vi "get path to CoreEngine dll.vi"() -> (6 "path to c_interface_calib_vc100.dll":path, 8 "path to c_interface_vc100.dll":path, 10 "path to imoptif":path, 12 "Release/Debug":string)   [LabVIEW 2020]
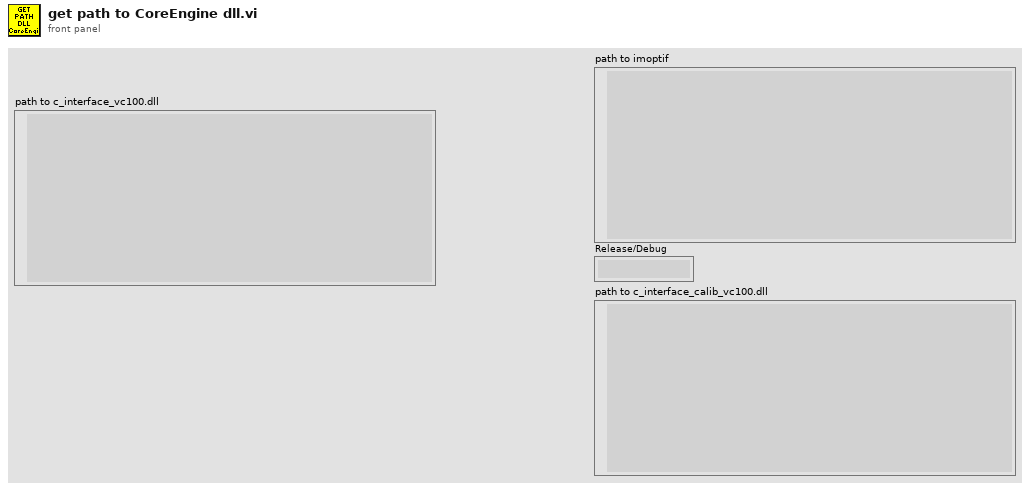
[diagram p1: front panel]
types:
  T1 = enum32{"invalid app kind", "Development System", "Run Time System", "Student Edition", "Embedded LabVIEW", "Evaluation", "Custom"}
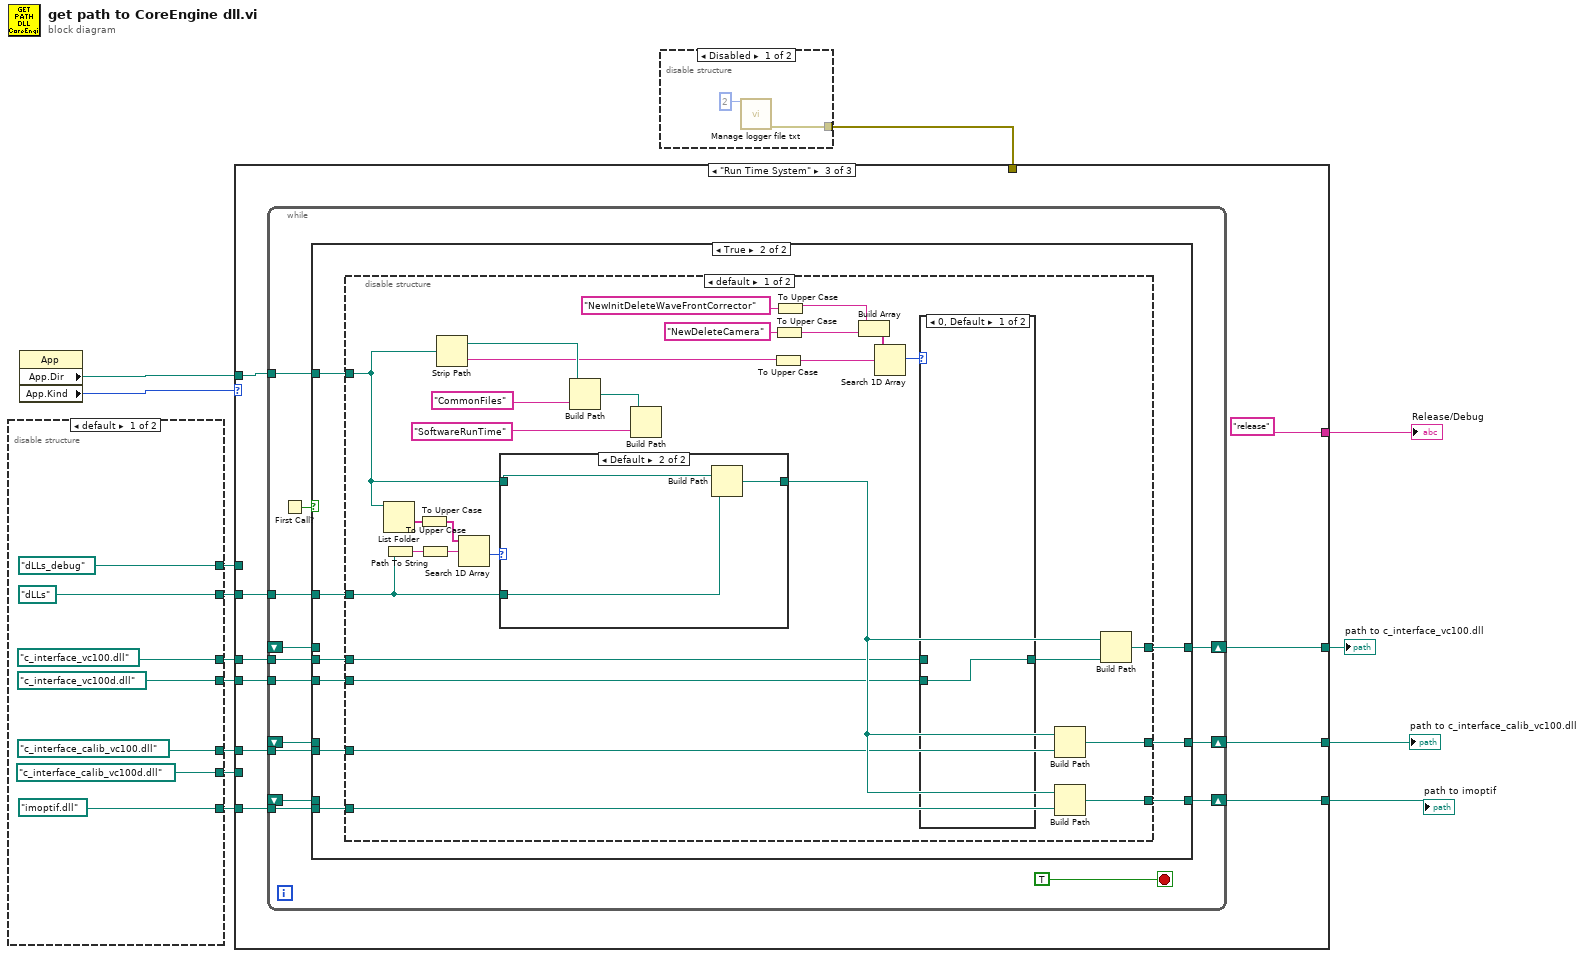
[diagram p0: block diagram]
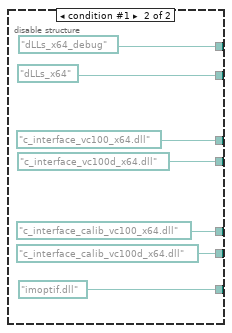
[diagram p3: hidden frame]
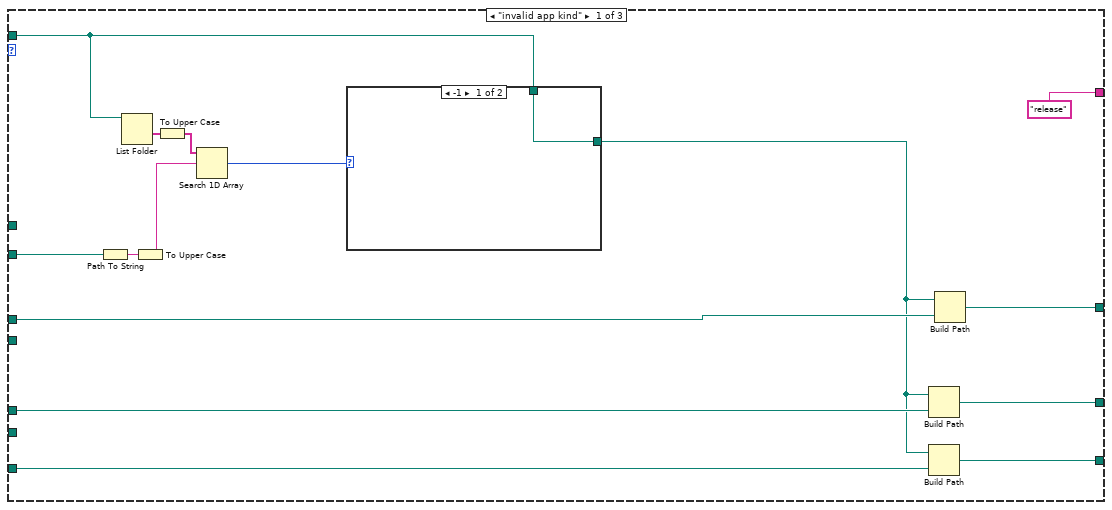
[diagram p4: hidden frame]
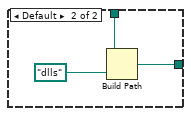
[diagram p5: hidden frame]
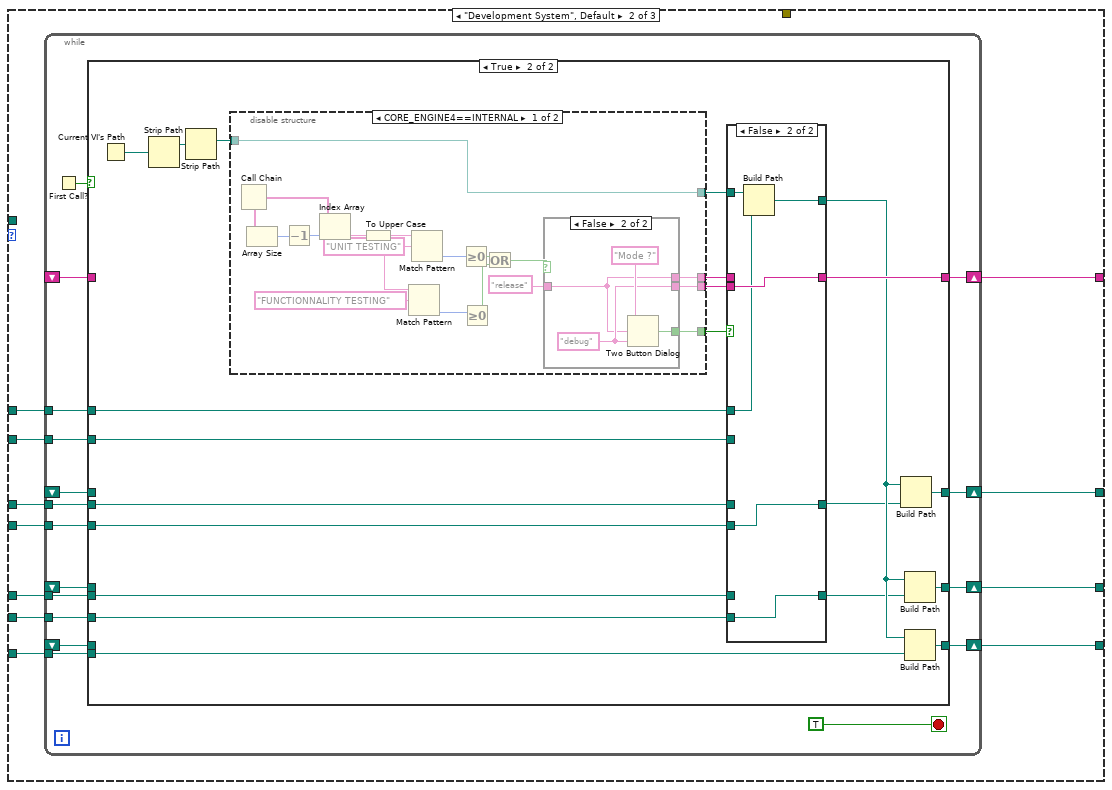
[diagram p6: hidden frame]
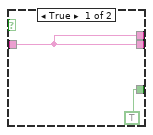
[diagram p8: hidden frame]
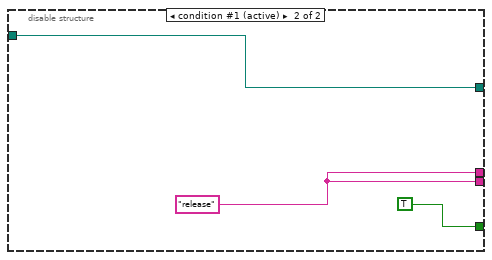
[diagram p9: hidden frame]
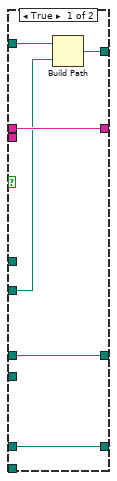
[diagram p10: hidden frame]
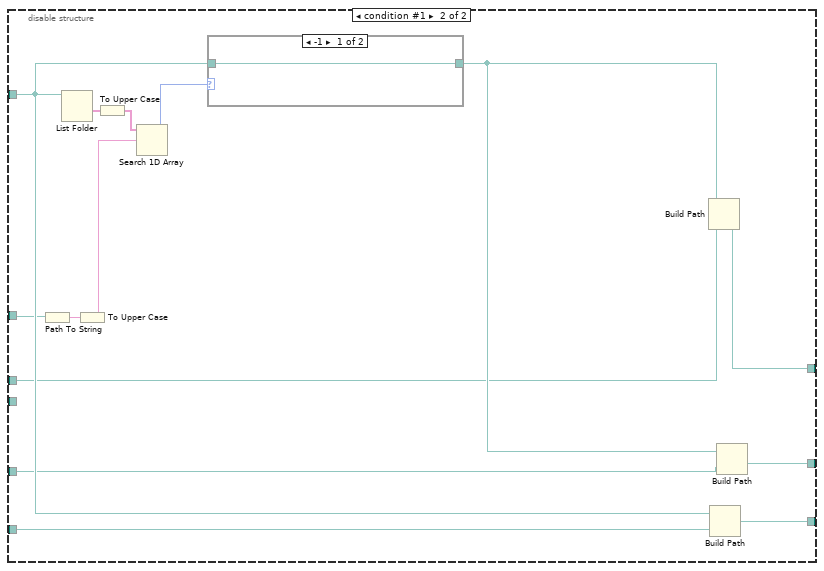
[diagram p14: hidden frame]
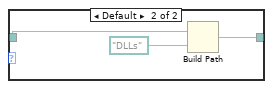
[diagram p15: hidden frame]
diagram:
  n1 = disable-structure shown="default" {
    disable-tunnel: [path "imoptif.dll" ("path in") path "imoptif.dll" ("path in")] -> w13
    disable-tunnel: [path "c_interface_vc100.dll" ("path in") path "c_interface_vc100_x64.dll" ("path in")] -> w8
    disable-tunnel: [path "c_interface_calib_vc100.dll" ("path in") path "c_interface_calib_vc100_x64.dll" ("path in")] -> w7
    disable-tunnel: [path "dLLs" ("path in") path "dLLs_x64" ("path in")] -> w5
    disable-tunnel: [path "dLLs_debug" ("path in") path "dLLs_x64_debug" ("path in")] -> w4
    disable-tunnel: [path "c_interface_vc100d.dll" ("path in") path "c_interface_vc100d_x64.dll" ("path in")] -> w3
    disable-tunnel: [path "c_interface_calib_vc100d.dll" ("path in") path "c_interface_calib_vc100d_x64.dll" ("path in")] -> w2
    frame condition #0 (active) {
    }
    frame condition #1 {
    }
  }
  n2 = property class="App"() -> ("App.Dir"=w10:path, "App.Kind"=w14:T1)  [unwired: 2 in, 2 out]
  n3 = disable-structure shown="Disabled" {
    disable-tunnel: [w29 _] -> w1
    frame Disabled {
      n4 = call "Manage logger file txt.vi"("length"=2) -> ("error out"=w29:errorcluster)  [unwired: 14 in]
    }
    frame Enabled {
    }
  }
  n5 = case shown="\"Run Time System\"" w14 {
    tunnel: [w45 w59 w150] -> w9
    tunnel: w10 -> [w41 _ w147]
    tunnel: w13 -> [w44 w58 w149]
    tunnel: [w43 w57 w148] -> w12
    tunnel: ["release" ("T button name (\"OK\")") w60 "release" ("T button name (\"OK\")")] -> w11
    tunnel: w8 -> [w37 w56 w144]
    tunnel: w7 -> [w36 w55 w143]
    tunnel: [w34 w54 w145] -> w6
    tunnel: w5 -> [w31 w53 w142]
    tunnel: w4 -> [_ w52 _]
    tunnel: w3 -> [_ w51 w141]
    tunnel: w2 -> [_ w50 _]
    tunnel: w1 -> [_ _ _]
    frame "invalid app kind" {
      n6 = Path To String(path=w31) -> (string=w33:string)
      n7 = List Folder(path=w41) -> (folder names=w40:string[])  [unwired: 3 in, 3 out]
      n8 = To Upper Case(1:w33) -> (0:w32:string)
      n9 = To Upper Case(1:w40) -> (0:w38:string[])
      n10 = Search 1D Array(1D array=w38, element=w32) -> (index of element=w39:i32)  [unwired: 1 in]
      n11 = case shown="-1" w39 {
        tunnel: [w46 w48] -> w35
        tunnel: w41 -> [w46 w47]
        frame -1 {
        }
        frame Default {
          n12 = Build Path(base path=w47, name or relative path=path "dlls" ("path in")) -> (appended path=w48:path)
        }
      }
      n13 = Build Path(base path=w35, name or relative path=w36) -> (appended path=w34:path)
      n14 = Build Path(base path=w35, name or relative path=w44) -> (appended path=w43:path)
      n15 = Build Path(base path=w35, name or relative path=w37) -> (appended path=w45:path)
    }
    frame "Development System", Default {
      n16 = while {
        shift-right: [w76] -> w59
        shift-left: _ -> [w75]
        shift-right: [w73] -> w60
        shift-left: _ -> [w72]
        shift-right: [w70] -> w57
        shift-left: _ -> [w69]
        tunnel: w58 -> [w71]
        tunnel: w56 -> [w68]
        tunnel: w55 -> [w67]
        shift-right: [w66] -> w54
        shift-left: _ -> [w65]
        tunnel: w53 -> [w64]
        tunnel: w52 -> [w63]
        tunnel: w51 -> [w62]
        tunnel: w50 -> [w61]
        stop <- TRUE stop-if-true
        n17 = First Call?() -> (First Call?: T/F=w77:bool)
        n18 = case shown="True" w77 {
          tunnel: [w81 w98] -> w76
          tunnel: w75 -> [w81 _]
          tunnel: [w80 w100] -> w73
          tunnel: w72 -> [w80 _]
          tunnel: w71 -> [_ w96]
          tunnel: [w79 w97] -> w70
          tunnel: w69 -> [w79 _]
          tunnel: w68 -> [_ w87]
          tunnel: w67 -> [_ w84]
          tunnel: [w78 w93] -> w66
          tunnel: w65 -> [w78 _]
          tunnel: w64 -> [_ w89]
          tunnel: w63 -> [_ w88]
          tunnel: w62 -> [_ w85]
          tunnel: w61 -> [_ w82]
          frame False {
          }
          frame True {
            n19 = Current VI's Path() -> (path=w94:path)
            n20 = Strip Path(path=w94) -> (stripped path=w95:path)  [unwired: 1 out]
            n21 = Strip Path(path=w95) -> (stripped path=w90:path)  [unwired: 1 out]
            n22 = disable-structure shown="CORE_ENGINE4==INTERNAL" {
              disable-tunnel: [w119 TRUE ("T button?")] -> w102
              disable-tunnel: [w118 w127] -> w101
              disable-tunnel: [w117 w127] -> w99
              disable-tunnel: [w103 w126] -> w92
              disable-tunnel: w90 -> [w103 w126]
              frame condition #0 {
                n23 = Call Chain() -> (call chain=w116:string[])
                n24 = Array Size(array=w116) -> (size(s)=w115:i32)
                n25 = Decrement(x=w115) -> (x-1=w114:i32)
                n26 = Index Array(array=w116, index=w114) -> (element=w113:string)
                n27 = To Upper Case(1:w113) -> (0:w110:string)
                n28 = Match Pattern(string=w110, regular expression="FUNCTIONNALITY TESTING") -> (offset past match=w107:i32)  [unwired: 1 in, 3 out]
                n29 = Match Pattern(string=w110, regular expression="UNIT TESTING") -> (offset past match=w108:i32)  [unwired: 1 in, 3 out]
                n30 = Greater Or Equal To 0?(x=w108) -> (x >= 0?=w106:bool)
                n31 = Greater Or Equal To 0?(x=w107) -> (x >= 0?=w105:bool)
                n32 = Or(x=w106, y=w105) -> (x .or. y?=w104:bool)
                n33 = case shown="False" w104 {
                  tunnel: [TRUE ("T button?") w125] -> w119
                  tunnel: [w121 w122] -> w118
                  tunnel: [w121 w123] -> w117
                  tunnel: "release" ("T button name (\"OK\")") -> [w121 w122]
                  frame True {
                  }
                  frame False {
                    w123 = "debug" ("F button name (\"Cancel\")")
                    n34 = Two Button Dialog(message="Mode ?", 1:w123, 2:w122) -> (T button?=w125:bool)
                  }
                }
              }
              frame condition #1 (active) {
                w127 = "release" ("T button name (\"OK\")")
              }
            }
            n35 = case shown="False" w102 {
              tunnel: [w134 w140] -> w100
              tunnel: w101 -> [w134 _]
              tunnel: w99 -> [_ w140]
              tunnel: w92 -> [w133 w139]
              tunnel: [w132 w138] -> w91
              tunnel: w89 -> [w131 _]
              tunnel: w88 -> [_ w137]
              tunnel: w87 -> [w130 _]
              tunnel: [w130 w136] -> w86
              tunnel: w85 -> [_ w136]
              tunnel: w84 -> [w129 _]
              tunnel: [w129 w135] -> w83
              tunnel: w82 -> [_ w135]
              frame True {
                n36 = Build Path(base path=w133, name or relative path=w131) -> (appended path=w132:path)
              }
              frame False {
                n37 = Build Path(base path=w139, name or relative path=w137) -> (appended path=w138:path)
              }
            }
            n38 = Build Path(base path=w91, name or relative path=w86) -> (appended path=w98:path)
            n39 = Build Path(base path=w91, name or relative path=w83) -> (appended path=w93:path)
            n40 = Build Path(base path=w91, name or relative path=w96) -> (appended path=w97:path)
          }
        }
      }
    }
    frame "Run Time System" {
      n41 = while {
        shift-right: [w163] -> w150
        shift-left: _ -> [w162]
        shift-right: [w159] -> w148
        shift-left: _ -> [w158]
        tunnel: w149 -> [w160]
        tunnel: w147 -> [w157]
        shift-right: [w154] -> w145
        shift-left: _ -> [w153]
        tunnel: w144 -> [w156]
        tunnel: w143 -> [w155]
        tunnel: w142 -> [w152]
        tunnel: w141 -> [w151]
        stop <- TRUE stop-if-true
        n42 = First Call?() -> (First Call?: T/F=w164:bool)
        n43 = case shown="True" w164 {
          tunnel: [w167 w176] -> w163
          tunnel: w162 -> [w167 _]
          tunnel: w160 -> [_ w174]
          tunnel: [w166 w173] -> w159
          tunnel: w158 -> [w166 _]
          tunnel: w157 -> [_ w175]
          tunnel: w156 -> [_ w172]
          tunnel: w155 -> [_ w171]
          tunnel: [w165 w170] -> w154
          tunnel: w153 -> [w165 _]
          tunnel: w152 -> [_ w169]
          tunnel: w151 -> [_ w168]
          frame False {
          }
          frame True {
            n44 = disable-structure shown="default" {
              disable-tunnel: [w204 w224] -> w176
              disable-tunnel: w175 -> [w198 w220]
              disable-tunnel: w174 -> [w200 w219]
              disable-tunnel: [w199 w218] -> w173
              disable-tunnel: w172 -> [w177 w214]
              disable-tunnel: w171 -> [w192 w215]
              disable-tunnel: [w191 w217] -> w170
              disable-tunnel: w169 -> [w182 w212]
              disable-tunnel: w168 -> [w179 _]
              frame condition #0 (active) {
                n45 = List Folder(path=w198) -> (folder names=w203:string[])  [unwired: 3 in, 3 out]
                n46 = Path To String(path=w182) -> (string=w181:string)
                n47 = To Upper Case(1:w203) -> (0:w202:string[])
                n48 = To Upper Case(1:w181) -> (0:w180:string)
                n49 = Strip Path(path=w198) -> (stripped path=w197:path, name=w190:string)
                n50 = Search 1D Array(1D array=w202, element=w180) -> (index of element=w201:i32)  [unwired: 1 in]
                n51 = case shown="Default" w201 {
                  tunnel: [w207 w210] -> w193
                  tunnel: w198 -> [w207 w209]
                  tunnel: w182 -> [_ w208]
                  frame -1 {
                  }
                  frame Default {
                    n52 = Build Path(base path=w209, name or relative path=w208) -> (appended path=w210:path)
                  }
                }
                n53 = Build Path(base path=w197, name or relative path="CommonFiles" ("element")) -> (appended path=w195:path)
                n54 = Build Path(base path=w195, name or relative path="SoftwareRunTime" ("element")) -> ()  [unwired: 1 out]
                n55 = To Upper Case(1:w190) -> (0:w184:string)
                n56 = To Upper Case(1:"NewDeleteCamera" ("element")) -> (0:w186:string)
                n57 = To Upper Case(1:"NewInitDeleteWaveFrontCorrector" ("element")) -> (0:w187:string)
                n58 = Build Array(w187, w186) -> (w185:string[])
                n59 = Search 1D Array(1D array=w185, element=w184) -> (index of element=w183:i32)  [unwired: 1 in]
                n60 = case shown="0, Default" w183 {
                  tunnel: [w205 w206] -> w178
                  tunnel: w179 -> [w205 _]
                  tunnel: w177 -> [_ w206]
                  frame 0, Default {
                  }
                  frame -1 {
                  }
                }
                n61 = Build Path(base path=w193, name or relative path=w192) -> (appended path=w191:path)
                n62 = Build Path(base path=w193, name or relative path=w200) -> (appended path=w199:path)
                n63 = Build Path(base path=w193, name or relative path=w178) -> (appended path=w204:path)
              }
              frame condition #1 {
                n64 = Path To String(path=w212) -> (string=w213:string)
                n65 = List Folder(path=w220) -> (folder names=w223:string[])  [unwired: 3 in, 3 out]
                n66 = To Upper Case(1:w213) -> (0:w211:string)
                n67 = To Upper Case(1:w223) -> (0:w222:string[])
                n68 = Search 1D Array(1D array=w222, element=w211) -> (index of element=w221:i32)  [unwired: 1 in]
                n69 = case shown="-1" w221 {
                  tunnel: [w225 w227] -> w216
                  tunnel: w220 -> [w225 w226]
                  frame -1 {
                  }
                  frame Default {
                    n70 = Build Path(base path=w226, name or relative path=path "DLLs" ("path in")) -> (appended path=w227:path)
                  }
                }
                n71 = Build Path(base path=w216, name or relative path=w214) -> (appended path=w224:path)
                n72 = Build Path(base path=w220, name or relative path=w219) -> (appended path=w218:path)
                n73 = Build Path(base path=w216, name or relative path=w215) -> (appended path=w217:path)
              }
            }
          }
        }
      }
    }
  }
  "path to c_interface_vc100.dll" <- w9
  "path to imoptif" <- w12
  "Release/Debug" <- w11
  "path to c_interface_calib_vc100.dll" <- w6
